vi "read_spectra_new_Flash.vi"() -> (0 "correction":dbl[](array[numeric]))   [LabVIEW 2022 SP3]
panel:
  out "Waveform Graph 2":dbl[](graph)
  out "Read_data":u8[](array[numeric])
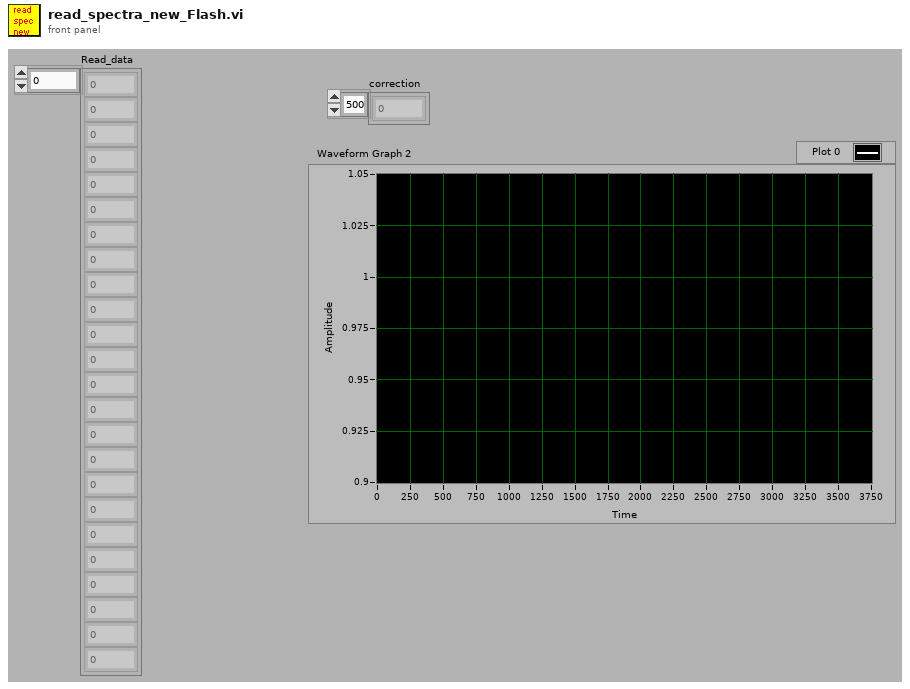
[diagram p1: front panel]
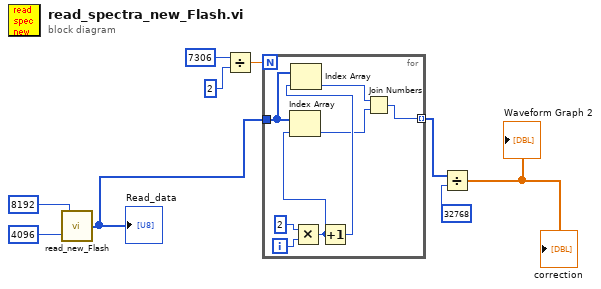
[diagram p0: block diagram]
diagram:
  n1 = call "read_new_Flash.vi"("address (3 bytes)"=u32 4096, "read_bytes"=u64 8192) -> ("Read_data"=w1:u8[])
  "Read_data" <- w1
  n2 = Divide(x=7306 ("dimension size"), y=2) -> (x/y=w7:dbl)
  n3 = for {
    N: w7 -> [_]
    tunnel: w1 -> [w14]
    tunnel: [w10] -> w3 mode=indexing
    i -> [w17]
    n4 = Multiply(x=2, y=w17) -> (x*y=w15:i32)
    n5 = Index Array(array=w14, index=w15) -> (element=w12:u8)
    n6 = Increment(x=w15) -> (x+1=w13:i32)
    n7 = Index Array(array=w14, index=w13) -> (element=w11:u8)
    n8 = Join Numbers(hi=w11, lo=w12) -> ((hi.lo)=w10:u16)
  }
  n9 = Divide(x=w3, y=u16 32768) -> (x/y=→"Waveform Graph 2" →"correction":dbl[])
